vi "ByRef In-Place Rebundle.vi"   [LabVIEW 2018]
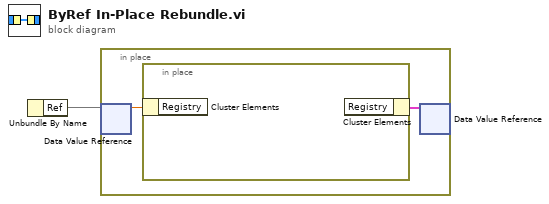
[diagram p0: block diagram]
diagram:
  n1 = Unbundle By Name() -> ("Ref"=w1)  [unwired: 1 in]
  n2 = in-place {
    n3 = in-place-dvr #1(w1) -> (w3:dbl)  [unwired: 1 out]
    n4 = in-place {
      n5 = in-place-cluster #2(w3) -> ()  [unwired: 1 out]
      n6 = in-place-cluster #2() -> (w2:cluster{})  [unwired: 1 in]
    }
    n7 = in-place-dvr #1(w2) -> ()  [unwired: 2 out]
  }
